vi "Detector Get Image.vi"(8 "error in (no error)":errorcluster, 10 "Observation":T1={"Priority"=0, "ID"="", "Observer"="", "Obj Name"="", "Obj Type"="", "RA and DEC String"={"RA"="HH:MM:SS.nnn", "DEC"="DEG:arcmin:arcsec.nn"}, "Filters"=[], "Integration Time"=0.0, "Observation Status"=enum."Error", "Offsets"={"RA"=0.0, "DEC"=0.0, "ROT"=0.0}, "Images"=0, "Dither Options"={"Dither"=enum."None", "Dither Radius"=0.0, "Dither Points"=0, "Dither Phase"=0.0, "B Offset"={"RA"=0.0, "DEC"=0.0}}, "Comment 1"="", "Comment 2"=""}, 11 "Detector Simulator in":refnum<class "Detector Simulator.lvclass">) -> (0 "error out":errorcluster, 1 "FITS Detector Settings":T8, 2 "Images":T9[](array[typedef]), 3 "Detector Simulator out":refnum<class "Detector Simulator.lvclass">, 4 "Message Log":string, 6 "Detector Files":T7)   [LabVIEW 2024, in "Detector Simulator.lvclass"]
uses:
  Detector Simulator.lvclass
  Detector Class/Detector Image typedef cluster.ctl
  RIMAS Observation Config.ctl
  Detector Class/Detector cluster Files.ctl
  typedefs/CC cluster Observation.ctl
  Observation Queue/CC enum Observation Status.ctl
  Telescope/CC cluster Telescope Offsets.ctl
  typedefs/CC cluster Observation Dither Options.ctl
  typedefs/CC enum Dither Selection.ctl
  typedefs/CC cluster RA and DEC.ctl
  Detector Class/Detector Class.lvclass
  Detector Simulator.lvclass/Detector Simulator.ctl
panel:
  # "sec"
  # "sec"
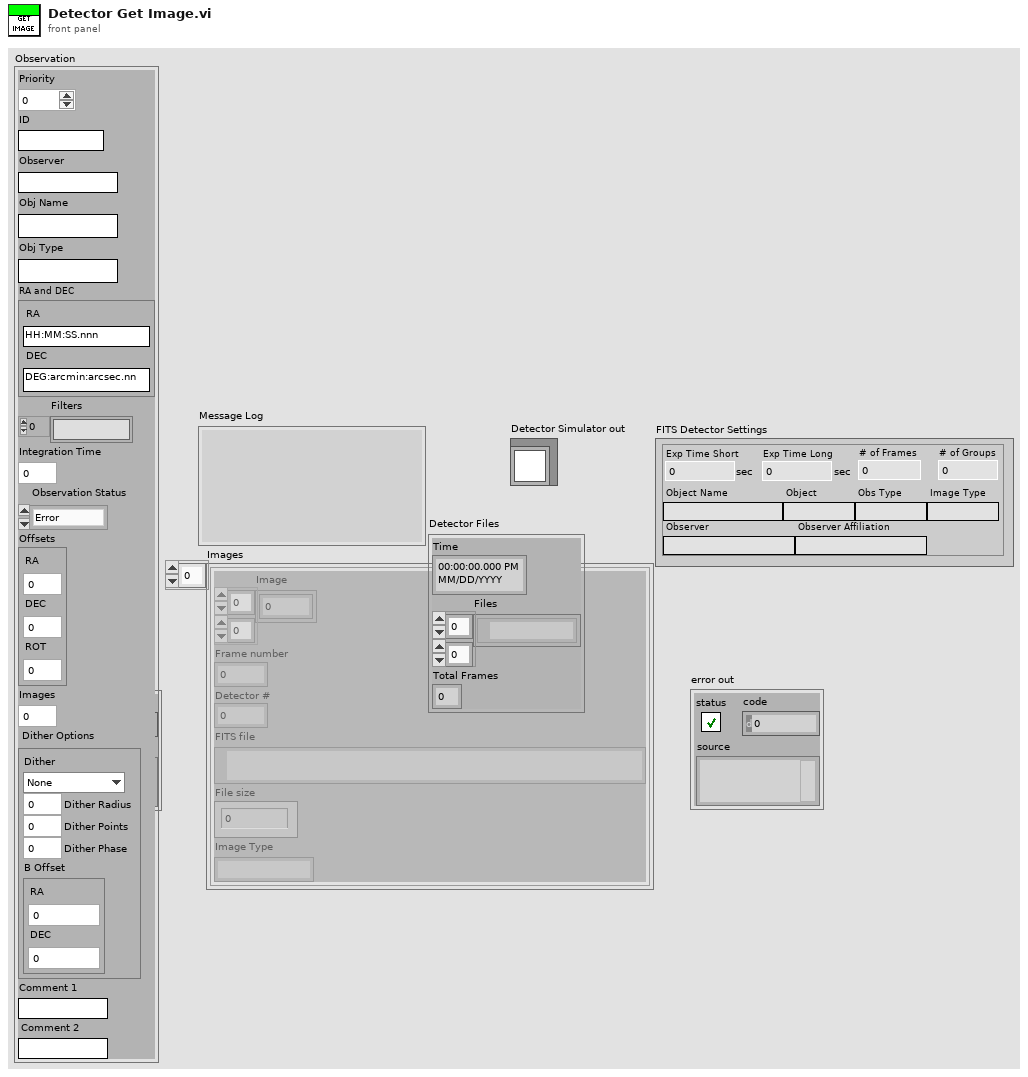
[diagram p1: front panel]
types:
  T1 = typedef "CC cluster Observation.ctl" = cluster{"Priority":i32, "ID":string, "Observer":string, "Obj Name":string, "Obj Type":string, "RA and DEC String":cluster{"RA":string, "DEC":string}, "Filters":string[], "Integration Time":dbl, "Observation Status":T2, "Offsets":T3, "Images":i32, "Dither Options":T4, "Comment 1":string, "Comment 2":string}
  T2 = typedef "CC enum Observation Status.ctl" = enum16{"Ready", "Running", "Done", "Error"}
  T3 = typedef "CC cluster Telescope Offsets.ctl" = cluster{"RA":dbl, "DEC":dbl, "ROT":dbl}
  T4 = typedef "CC cluster Observation Dither Options.ctl" = cluster{"Dither":T5, "Dither Radius":dbl, "Dither Points":i32, "Dither Phase":dbl, "B Offset":T6}
  T5 = typedef "CC enum Dither Selection.ctl" = enum16{"None", "Circle", "Random", "ABBA"}
  T6 = typedef "CC cluster RA and DEC.ctl" = cluster{"RA":dbl, "DEC":dbl}
  T7 = typedef "Detector Class.lvclass/Detector cluster Files.ctl" = cluster{"Time":timestamp, "Files":path[][], "Total Frames":i32}
  T8 = typedef "RIMAS Observation Config.ctl" = cluster{"Exp Time Short":dbl, "# of Frames":dbl, "Exp Time Long":dbl, "# of Groups":dbl, "Object Name":string, "Object":string, "Obs Type":string, "Image Type":string, "Observer":string, "Observer Affiliation":string}
  T9 = typedef "Detector Class.lvclass/Detector Image typedef cluster.ctl" = cluster{"Image":sgl[][], "Frame number":i32, "Detector #":u16, "FITS file":path, "File size":i64, "Image Type":string}
  T10 = typedef "RIMAS Detector Config.ctl" = cluster{"Detector":u16, "Offsets":u16[][], "Detector Computer":T11, "FITS hdr template0":path, "FITS hdr template1":path, "FITS Data File Path":path, "FITS Detector Settings":T8, "Sim Folder":path, "Integration Mode":T12, "Integration Time":dbl, "Frame Int Time":dbl}
  T11 = typedef "RIMAS Detector Server Config.ctl" = cluster{"Machine":string, "Password":string, "FITS File Path":string, "Port":u16, "Header Path":string, "Name":string}
  T12 = typedef "Detector enum Detector Integration Mode.ctl" = enum16{"Ramp", "CDS", "FOWLER2", "FOWLER4", "FOWLER8", "FOWLER16", "Raw"}
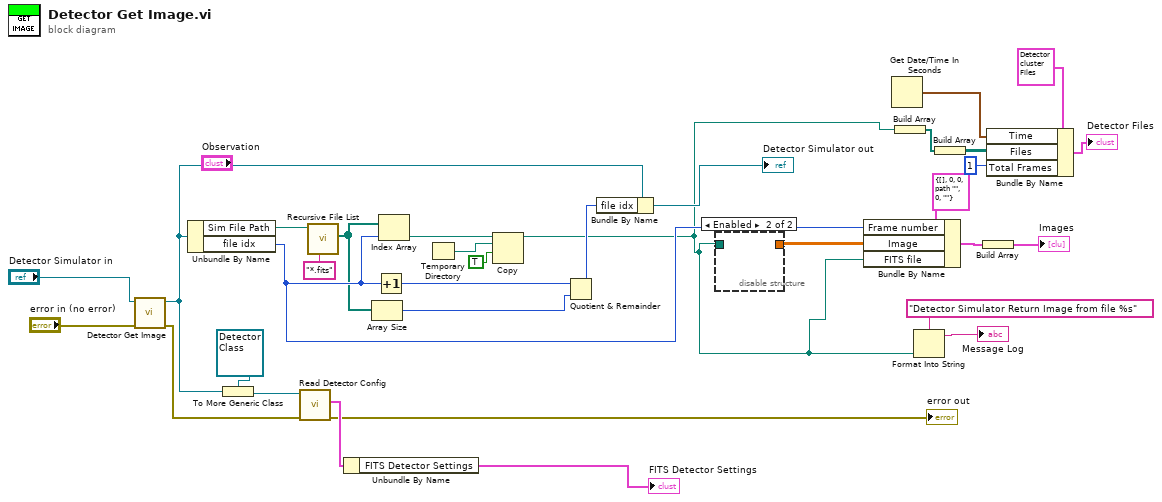
[diagram p0: block diagram]
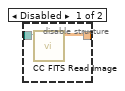
[diagram p2: hidden frame]
diagram:
  n1 = call-parent "Detector Get Image.vi"("error in (no error)"="error in (no error)", "Detector Class in"="Detector Simulator in") -> ("error out"=w18:errorcluster, "Detector Class out"=w22:refnum<class "Detector Simulator.lvclass">)  [unwired: 4 in, 4 out]
  n2 = Unbundle By Name(w22) -> ("Sim File Path"=w16:path, "file idx"=w26:i32)
  n3 = To More Generic Class(target class=refnum<class "Detector Class.lvclass"> refnum ("Detector Class.lvclass"), reference=w22) -> (generic class reference=w20:refnum<class "Detector Class.lvclass">)
  n4 = call-dynamic "Read Detector Config.vi"("error in (no error)"=w18, "Detector Class in"=w20) -> ("error out"=→"error out":errorcluster, "Detector Config"=w19:T10)  [unwired: 7 in, 1 out]
  n5 = call <vilib>:"Recursive File List.vi"("pattern"="*.fits", "Folder Path"=w16) -> ("All Files in Dir"=w14:path[])  [unwired: 5 in, 4 out]
  n6 = Unbundle By Name(w19) -> ("FITS Detector Settings"=→"FITS Detector Settings":T8)
  n7 = Array Size(array=w14) -> (size(s)=w30:i32)
  n8 = Increment(x=w26) -> (x+1=w31:i32)
  n9 = Index Array(array=w14, index=w26) -> (element=w2:path)
  n10 = Temporary Directory() -> (w4:path)
  n11 = Copy(9:TRUE ("overwrite (F)"), 10:w4, 11:w2) -> (3:w1:path)  [unwired: 2 in, 2 out]
  n12 = Quotient & Remainder(x=w31, y=w30) -> (x-y*floor(x/y)=w27:i32)  [unwired: 1 out]
  n13 = Bundle By Name(cluster=w22, "file idx"=w27) -> (→"Detector Simulator out":refnum<class "Detector Simulator.lvclass">)
  n14 = disable-structure shown="Enabled" {
    disable-tunnel: [w35 _] -> w12
    disable-tunnel: w1 -> [w34 _]
    frame Disabled {
      n15 = call "CC FITS Read Image.vi"("FITS File Path"=w34) -> ("Image"=w35:sgl[][])  [unwired: 9 in, 1 out]
    }
    frame Enabled {
    }
  }
  n16 = Bundle By Name(cluster=T9 {"Image"=[], "Frame number"=0, "Detector #"=0, "FITS file"=path "", "File size"=0, "Image Type"=""} ("Image Data"), "Frame number"=w26, "Image"=w12, "FITS file"=w1) -> (w25:T9)
  n17 = Get Date/Time In Seconds() -> (seconds since 1Jan1904=w8:timestamp)
  n18 = Build Array(w1) -> (w10:path[])
  n19 = Format Into String(format string="Detector Simulator Return Image from file %s", w1) -> (resulting string=→"Message Log":string)  [unwired: 2 in, 1 out]
  n20 = Build Array(w10) -> (w9:path[][])
  n21 = Build Array(w25) -> (→"Images":T9[])
  n22 = Bundle By Name(cluster=T7 {"Time"=timestamp(0 s since 1904-01-01), "Files"=[], "Total Frames"=0} ("Detector Files"), "Time"=w8, "Files"=w9, "Total Frames"=1) -> (→"Detector Files":T7)
